vi "Set Conductivity Range.vi"(8 "error in (no error)":errorcluster, 9 "Range":T1, 10 "Channel":T2, 11 "EPU452 in":refnum<class "EPU452.lvclass">) -> (0 "error out":errorcluster, 2 "Response":string, 3 "EPU452 out":refnum<class "EPU452.lvclass">)   [LabVIEW 2018, in "EPU452.lvclass"]
uses:
  EPU452.lvclass
  Controls/Channels.ctl
  Controls/Conductivity Ranges.ctl
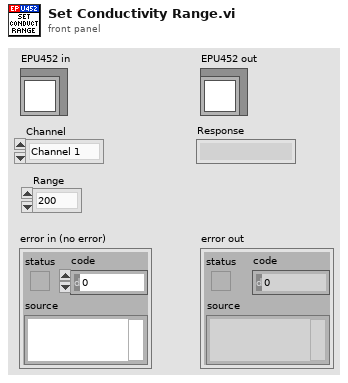
[diagram p1: front panel]
types:
  T1 = typedef "EPU452.lvclass/Conductivity Ranges.ctl" = enum16{"200", "20", "2", "0.2", "0.02", "0.002"}
  T2 = typedef "EPU452.lvclass/Channels.ctl" = enum16{"Channel 1", "Channel 2", "Channel 3", "Channel 4"}
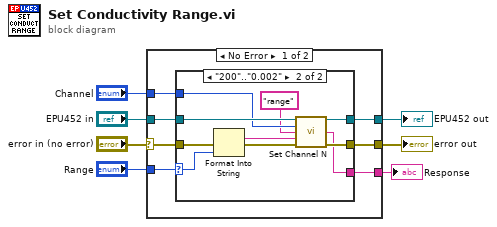
[diagram p0: block diagram]
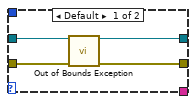
[diagram p2: hidden frame]
diagram:
  n1 = case shown="No Error" "error in (no error)" {
    selector: "error in (no error)" -> [w12 w30]
    tunnel: [w9 w30] -> w6
    tunnel: [w10 w29] -> w4
    tunnel: "EPU452 in" -> [w14 w29]
    tunnel: "Channel" -> [w13 _]
    tunnel: "Range" -> [w11 _]
    tunnel: [w8 _] -> w1
    frame No Error {
      n2 = case shown="\"200\"..\"0.002\"" w11 {
        selector: w11 -> [_ w23]
        tunnel: w14 -> [w17 w28]
        tunnel: w13 -> [_ w27]
        tunnel: w12 -> [w18 w22]
        tunnel: [w16 w25] -> w10
        tunnel: [w15 w24] -> w9
        tunnel: [_ w19] -> w8
        frame Default {
          n3 = call "Out of Bounds Exception.vi"("error in (no error)"=w18, "EPU452 in"=w17) -> ("error out"=w15:errorcluster, "EPU452 out"=w16:refnum<class "EPU452.lvclass">)  [unwired: 8 in]
        }
        frame "200".."0.002" {
          n4 = Format Into String(error in=w22, w23) -> (resulting string=w20:string, error out=w21:errorcluster)  [unwired: 2 in]
          n5 = call "Set Channel N.vi"("EPU452 in"=w28, "Channel"=w27, "Function"="range", "Argument/s"=w20, "error in (no error)"=w21) -> ("EPU452 out"=w25:refnum<class "EPU452.lvclass">, "Response"=w19:string, "error out"=w24:errorcluster)  [unwired: 8 in]
        }
      }
    }
    frame Error {
    }
  }
  "error out" <- w6
  "EPU452 out" <- w4
  "Response" <- w1
